vi "Filter Control Clusters.vi"(8 "Error In":errorcluster, 11 "GObjects In":refnum<vi>[](array[refnum])) -> (0 "Error Out":errorcluster, 3 "GObjects Out":refnum<vi>[](array[refnum]))   [LabVIEW 2017]
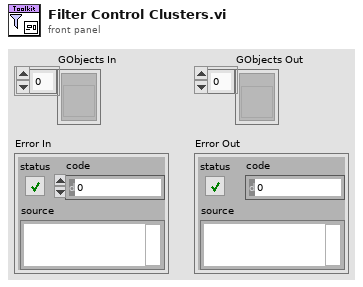
[diagram p1: front panel]
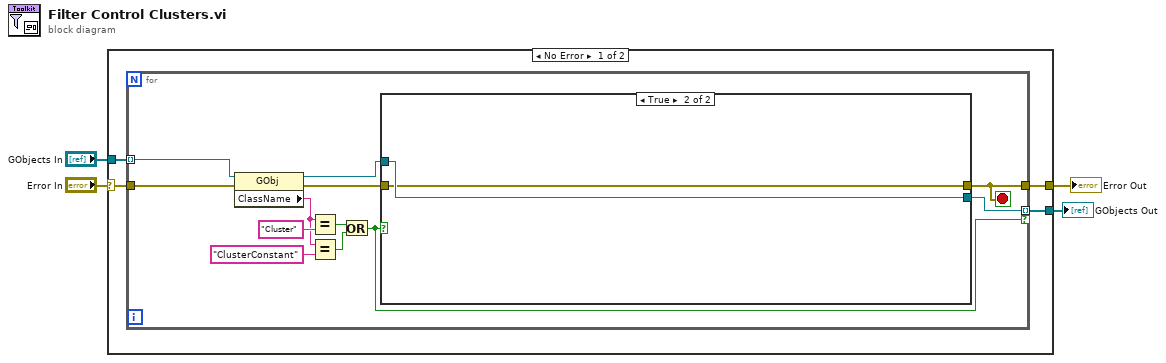
[diagram p0: block diagram]
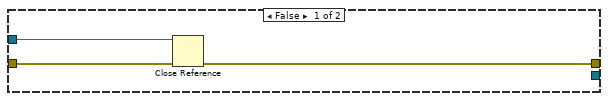
[diagram p2: hidden frame]
diagram:
  n1 = case shown="No Error" "Error In" {
    selector: "Error In" -> [w7 w26]
    tunnel: "GObjects In" -> [w8 _]
    tunnel: [w5 w26] -> w2
    tunnel: [w6 _] -> w1
    frame No Error {
      n2 = for {
        tunnel: w8 -> [w20] mode=indexing
        tunnel: w7 -> [w19]
        tunnel: [w15] -> w6 mode=indexing if=w9
        tunnel: [w10] -> w5
        stop <- w10 stop-if-true
        n3 = property class="GObj"(reference=w20, error in=w19) -> (reference out=w17:refnum<vi>, error out=w11:errorcluster, "ClassName"=w12:string)
        n4 = Equal?(x=w12, y="Cluster") -> (x = y?=w13:bool)
        n5 = Equal?(x=w12, y="ClusterConstant") -> (x = y?=w16:bool)
        n6 = Or(x=w13, y=w16) -> (x .or. y?=w9:bool)
        n7 = case shown="True" w9 {
          tunnel: w17 -> [w23 w25]
          tunnel: w11 -> [w22 w24]
          tunnel: [w21 w24] -> w10
          tunnel: [_ w25] -> w15
          frame False {
            n8 = Close Reference(reference=w23, error in (no error)=w22) -> (error out=w21:errorcluster)
          }
          frame True {
          }
        }
      }
    }
    frame Error {
    }
  }
  "Error Out" <- w2
  "GObjects Out" <- w1
